vi "updateCurrentOutputState.vi"(8 "error in (no error)":errorcluster, 9 "calibratedValues":dbl[](array[numeric]), 10 "channel_addresses":string[](array[string]), 11 "AnalogOutput in":refnum<class "AnalogOutput.lvclass">) -> (0 "error out":errorcluster, 3 "AnalogOutput out":refnum<class "AnalogOutput.lvclass">)   [LabVIEW 2011, in "Hardware.lvlib" / "Channels.lvlib" / "AnalogOutput.lvclass"]
uses:
  AnalogOutput.lvclass
  AnalogOutput.lvclass/AnalogOutput.ctl
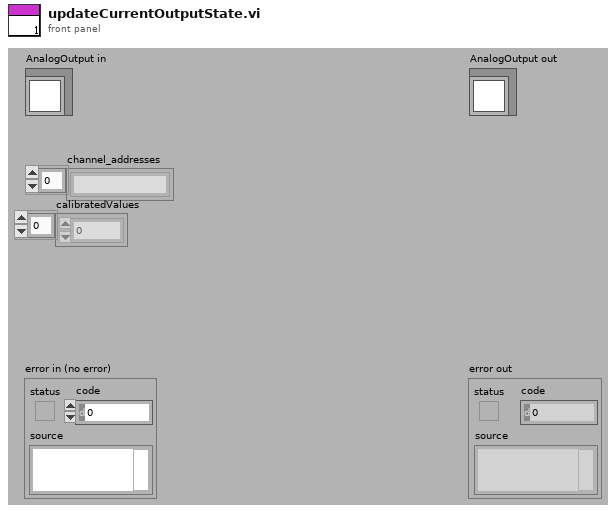
[diagram p1: front panel]
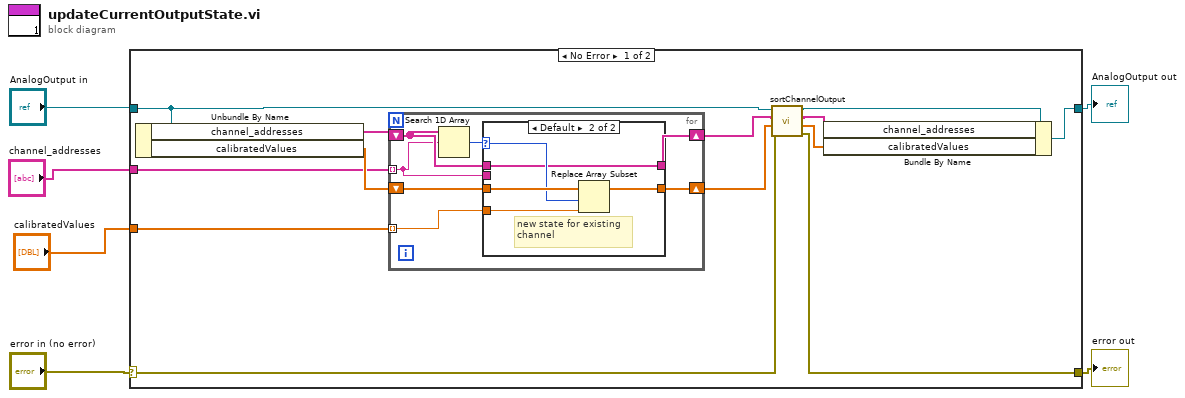
[diagram p0: block diagram]
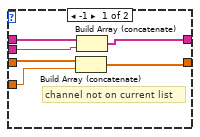
[diagram p2: hidden frame]
diagram:
  n1 = case shown="No Error" "error in (no error)" {
    selector: "error in (no error)" -> [w11 w39]
    tunnel: [w10 w39] -> w2
    tunnel: [w16 w38] -> w1
    tunnel: "AnalogOutput in" -> [w15 w38]
    tunnel: "channel_addresses" -> [w7 _]
    tunnel: "calibratedValues" -> [w18 _]
    frame No Error {
      n2 = Unbundle By Name(w15) -> ("channel_addresses"=w19:string[], "calibratedValues"=w17:dbl[])
      n3 = for {
        tunnel: w7 -> [w21] mode=indexing
        tunnel: w18 -> [w24] mode=indexing
        shift-right: [w23] -> w12
        shift-left: w17 -> [w25]
        shift-right: [w20] -> w13
        shift-left: w19 -> [w22]
        n4 = Search 1D Array(1D array=w22, element=w21) -> (index of element=w26:i32)  [unwired: 1 in]
        n5 = case shown="Default" w26 {
          selector: w26 -> [_ w35]
          tunnel: w25 -> [w32 w37]
          tunnel: w24 -> [w31 w36]
          tunnel: [w30 w34] -> w23
          tunnel: w22 -> [w29 w33]
          tunnel: w21 -> [w28 _]
          tunnel: [w27 w33] -> w20
          frame -1 {
            # "channel not on current list"
            n6 = Build Array (concatenate)(w32, w31) -> (w30:dbl[])
            n7 = Build Array (concatenate)(w29, w28) -> (w27:string[])
          }
          frame Default {
            # "new state for existing \nchannel"
            n8 = Replace Array Subset(array=w37, new element=w36, index=w35) -> (w34:dbl[])
          }
        }
      }
      n9 = call "sortChannelOutput.vi"("error in (no error)"=w11, "calibratedValues"=w12, "channel_addresses"=w13, "AnalogOutput in"=w15) -> ("error out"=w10:errorcluster, "calibratedValues out"=w9:dbl[], "channel_addresses out"=w8:string[], "AnalogOutput out"=w14:refnum<class "AnalogOutput.lvclass">)  [unwired: 4 in]
      n10 = Bundle By Name(cluster=w14, "channel_addresses"=w8, "calibratedValues"=w9) -> (w16:refnum<class "AnalogOutput.lvclass">)
    }
    frame Error {
    }
  }
  "error out" <- w2
  "AnalogOutput out" <- w1
